vi "Actor Core.vi"(8 "error in":errorcluster, 11 "IED in":refnum<class "IED.lvclass">) -> (0 "error out":errorcluster, 3 "Actor out":refnum<class "Actor.lvclass">)   [LabVIEW 2015, in "IED Actor.lvlib" / "IED.lvclass"]
doc: "(<B>Filename</B>: Actor Framework.lvlib:Actor.lvclass:Actor Core.vi)\n\nReceives messages to the actor, reacts to them, and initiates any error handling that may shut the actor down.\n\nDescendant classes may override this VI to append parallel tasks for the actor to complete while it handles messages. Overrides use the Call Parent Method node."
uses:
  IED.lvclass
  <vilib>/ActorFramework/Actor/Actor.lvclass
  <vilib>/ActorFramework/Actor/Actor.lvclass/Actor.ctl
  IED.lvclass/IED.ctl
  <vilib>/NI/Tools/Keyed Array/Map String.vi
  <vilib>/NI/Tools/String/Get Case Matching.vi
  <vilib>/Modbus/master/Modbus Master.lvclass
  <vilib>/NI/Tools/Keyed Array/Tools_KeyedArray.lvlib
  Utilities/Message Strings.llb/Message String Utilities.lvlib
  IED Messages/Store Value/Store Value Msg.lvclass
  Utilities/Modbus Data Conversion.llb/Modbus Data Conversion.lvlib
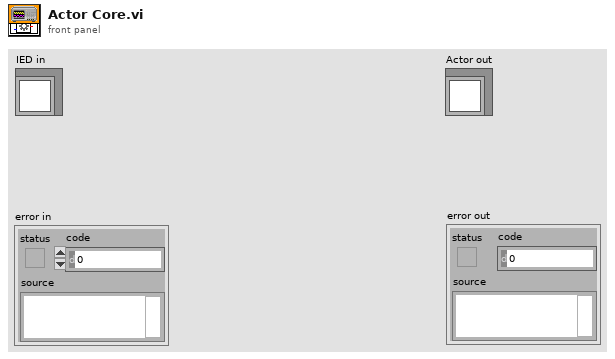
[diagram p1: front panel]
types:
  T1 = typedef "Tools_KeyedArray.lvlib/KeyedArray.ctl" = cluster{"keys":string[], "values":string[]}
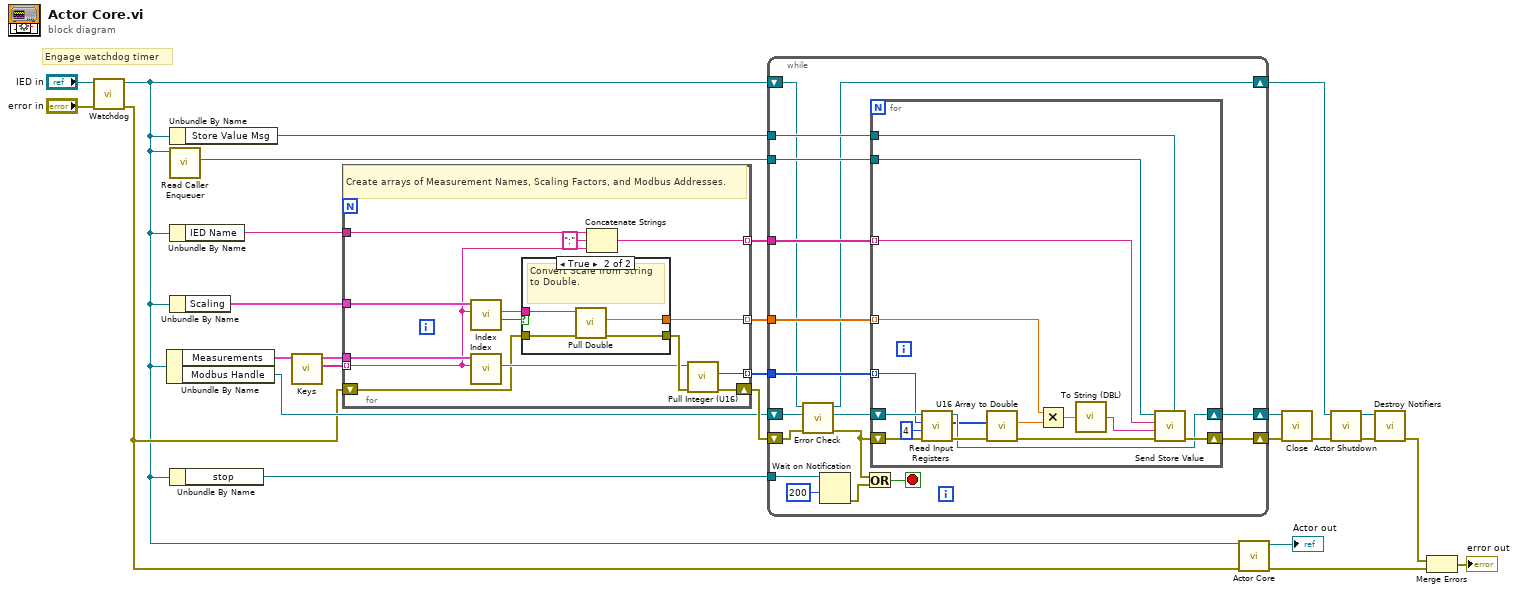
[diagram p0: block diagram]
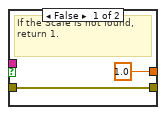
[diagram p2: hidden frame]
diagram:
  # "Engage watchdog timer"
  n1 = call "Watchdog.vi"("error in (no error)"="error in", "IED in"="IED in") -> ("error out"=w8:errorcluster, "IED out"=w5:refnum<class "IED.lvclass">)  [unwired: 8 in]
  n2 = Unbundle By Name(w5) -> ("Measurements"=w12:T1, "Modbus Handle"=w9:refnum<class "Modbus Master.lvclass">)
  n3 = Unbundle By Name(w5) -> ("Store Value Msg"=w24:refnum<class "Store Value Msg.lvclass">)
  n4 = call <vilib>:"Read Caller Enqueuer.vi"("Actor"=w5) -> ("Caller Enqueuer"=w23:refnum<class "Message Enqueuer.lvclass">)  [unwired: 10 in]
  n5 = Unbundle By Name(w5) -> ("IED Name"=w16:string)
  n6 = Unbundle By Name(w5) -> ("Scaling"=w17:T1)
  n7 = Unbundle By Name(w5) -> ("stop"=w11:refnum<notifier>)
  n8 = call <vilib>:"Keys.vi"("array in"=w12) -> ("keys"=w19:string[], "duplicate array"=w18:T1)  [unwired: 5 in]
  n9 = for {
    tunnel: w19 -> [w32] mode=indexing
    tunnel: w18 -> [w33]
    tunnel: w17 -> [w34]
    shift-right: [w37] -> w10
    shift-left: w8 -> [w36]
    tunnel: w16 -> [w35]
    tunnel: [w31] -> w13 mode=indexing
    tunnel: [w30] -> w14 mode=indexing
    tunnel: [w29] -> w15 mode=indexing
    # "Create arrays of Measurement Names, Scaling Factors, and Modbus Addresses."
    n10 = call <vilib>:"Index.vi"("key"=w32, "array in"=w34) -> ("valid key"=w28:bool, "value"=w39:string)  [unwired: 3 in, 1 out]
    n11 = call <vilib>:"Index.vi"("key"=w32, "array in"=w33) -> ("value"=w38:string)  [unwired: 3 in, 2 out]
    n12 = case shown="True" w28 {
      tunnel: [w43 w47] -> w40
      tunnel: w39 -> [_ w46]
      tunnel: w36 -> [w43 w45]
      tunnel: [1.0 ("Double out") w44] -> w30
      frame False {
        # "If the Scale is not found, return 1."
      }
      frame True {
        # "Convert Scale from String to Double."
        n13 = call "Pull Double.vi"("error in (no error)"=w45, "String in"=w46) -> ("error out"=w47:errorcluster, "Double out"=w44:dbl)  [unwired: 7 in, 1 out]
      }
    }
    n14 = Concatenate Strings(w35, ":" ("string"), w32) -> (w29:string)
    n15 = call "Pull Integer (U16).vi"("error in (no error)"=w40, "String in"=w38) -> ("error out"=w37:errorcluster, "Integer out"=w31:u16)  [unwired: 7 in, 1 out]
  }
  n16 = while {
    tunnel: w11 -> [w63]
    tunnel: w24 -> [w61]
    tunnel: w23 -> [w60]
    shift-right: [w64] -> w21
    shift-left: w10 -> [w54]
    shift-right: [w59] -> w20
    shift-left: w9 -> [w50]
    tunnel: w15 -> [w57]
    tunnel: w14 -> [w56]
    tunnel: w13 -> [w55]
    shift-right: [w51] -> w4
    shift-left: w5 -> [w52]
    stop <- w58 stop-if-true
    n17 = call "Error Check.vi"("error in (no error)"=w54, "Modbus master in"=w50, "IED in"=w52) -> ("error out"=w53:errorcluster, "Modbus master out"=w49:refnum<class "Modbus Master.lvclass">, "IED out"=w51:refnum<class "IED.lvclass">)  [unwired: 6 in]
    n18 = Wait on Notification(notifier=w63, timeout in ms (-1)=200) -> (error out=w48:errorcluster)  [unwired: 2 in, 3 out]
    n19 = Or(x=w53, y=w48) -> (x .or. y?=w58:bool)
    n20 = for {
      tunnel: w61 -> [w76]
      tunnel: w60 -> [w77]
      shift-right: [w72] -> w64
      shift-left: w53 -> [w70]
      shift-right: [w71] -> w59
      shift-left: w49 -> [w79]
      tunnel: w57 -> [w69] mode=indexing
      tunnel: w56 -> [w68] mode=indexing
      tunnel: w55 -> [w67] mode=indexing
      n21 = call-dynamic "Read Input Registers.vi"("error in (no error)"=w70, "number of input registers"=u16 4, "starting address"=w67, "Modbus master in"=w79) -> ("error out"=w73:errorcluster, "register values"=w66:u16[], "Modbus master out"=w71:refnum<class "Modbus Master.lvclass">)  [unwired: 5 in]
      n22 = call "U16 Array to Double.vi"("U16 Array"=w66) -> ("Double"=w65:dbl)  [unwired: 10 in]
      n23 = Multiply(x=w68, y=w65) -> (x*y=w75:dbl)
      n24 = call "To String (DBL).vi"("Double in"=w75) -> ("String out"=w74:string)
      n25 = call "Send Store Value.vi"("Store Value Msg"=w76, "error in (no error)"=w73, "Value"=w74, "Key"=w69, "Message Enqueuer in"=w77) -> ("error out"=w72:errorcluster)  [unwired: 5 in, 1 out]
    }
  }
  n26 = call-parent "Actor Core.vi"("error in"=w8, "Actor in"=w5) -> ("error out"=w26:errorcluster, "Actor out"=→"Actor out":refnum<class "Actor.lvclass">)  [unwired: 8 in]
  n27 = call-dynamic "Close.vi"("error in (no error)"=w21, "Modbus master in"=w20) -> ("error out"=w2:errorcluster)  [unwired: 9 in]
  n28 = call "Actor Shutdown.vi"("error in (no error)"=w2, "IED in"=w4) -> ("error out"=w1:errorcluster, "IED out"=w3:refnum<class "IED.lvclass">)  [unwired: 8 in]
  n29 = call "Destroy Notifiers.vi"("error in (no error)"=w1, "IED in"=w3) -> ("error out"=w22:errorcluster)  [unwired: 8 in, 1 out]
  n30 = Merge Errors(w22, w26) -> (→"error out":errorcluster)
